vi "OPM.GetPower.vi"(8 "error in (no error)":errorcluster, 11 "PM in":refnum<class "OPM.ThorlabsPM400.lvclass">) -> (0 "error out":errorcluster, 2 "Power, W":dbl format="%#_13g", 3 "PM out":refnum<class "OPM.ThorlabsPM400.lvclass">)   [LabVIEW 2019, in "OPM.ThorlabsPM400.lvclass"]
uses:
  OPM.ThorlabsPM400.lvclass
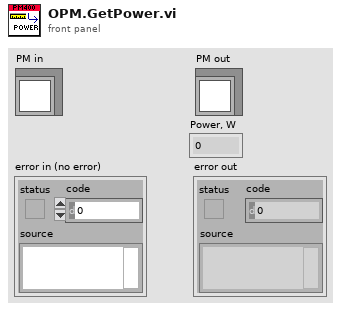
[diagram p1: front panel]
types:
  T1 = typedef "OPM.ThorlabsPM400.lvclass/Resource--Cluster.ctl" = cluster{"Instrument handle":refnum<visa-resource-name>}
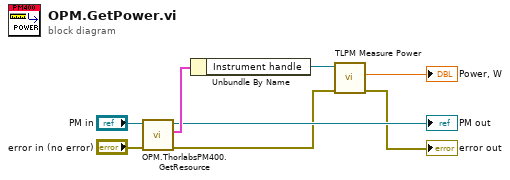
[diagram p0: block diagram]
diagram:
  n1 = call "OPM.ThorlabsPM400.GetResource.vi"("error in (no error)"="error in (no error)", "OPM.ThorlabsPM400 in"="PM in") -> ("error out"=w3:errorcluster, "Resource"=w6:T1, "OPM.ThorlabsPM400 out"=→"PM out":refnum<class "OPM.ThorlabsPM400.lvclass">)  [unwired: 7 in]
  n2 = Unbundle By Name(w6) -> ("Instrument handle"=w4:refnum<visa-resource-name>)
  n3 = call <instrlib>:"TLPM Measure Power.vi"("error in (no error)"=w3, "instrument handle"=w4) -> ("error out"=→"error out":errorcluster, "Power"=→"Power, W":dbl)  [unwired: 7 in, 1 out]
